vi "MPRL DDA.vi"() -> ()   [LabVIEW 2017]
uses:
  <vilib>/Platform/TimedLoop/XDataNode/timing_clust.ctl
  <vilib>/Platform/TimedLoop/XDataNode/nitl_modes.ctl
  <vilib>/Platform/TimedLoop/XDataNode/wakeup.ctl
  <vilib>/Analysis/Matrix/Datatypes/RealMatrix.ctl
  <vilib>/Analysis/_algsub.llb/Vector Norm Type.ctl
  <vilib>/Analysis/baseanly.llb/A x Vector.vi
  <vilib>/Analysis/baseanly.llb/Real A x B.vi
  <vilib>/Analysis/_algsub.llb/Real Vector Norm.vi
  <vilib>/Analysis/baseanly.llb/Outer Product.vi
  <vilib>/Analysis/baseanly.llb/Real Outer Product.vi
  <vilib>/robotics/Kinematics/Create Lie Group Matrix.vi
  <vilib>/Analysis/7linalg.llb/Create Special Matrix.vi
  <vilib>/Analysis/7linalg.llb/Create Special Real Matrix.vi
  <vilib>/Analysis/Matrix/Numeric/Multiply/Multiply.vi
  <vilib>/Analysis/Matrix/Numeric/Multiply/Multiply - RM,R.vi
  <vilib>/Analysis/Matrix/Numeric/Multiply/Multiply - R,RM.vi
  <vilib>/Analysis/Matrix/Numeric/Add/Add.vi
  <vilib>/Analysis/Matrix/Numeric/Add/Add - RM,RM.vi
  <vilib>/platform/TimedLoop/XDataNode/XDataNode.xnode
  <vilib>/robotics/Kinematics/NI_Kinematics.lvlib
  <vilib>/Analysis/NI_AALBase.lvlib
  <vilib>/Platform/TimedLoop/XDataNode/XDNodeRunTimeDep.lvlib
  <vilib>/Native 3D Graph/xcontrol/3DPC_SurfacePlot.xctl
  <vilib>/Analysis/Matrix/NI_Matrix.lvlib
  <vilib>/Analysis/NI_AALPro.lvlib
  <vilib>/Native 3D Graph/classes/Base Datatype.lvclass
panel:
  out "flag":bool
  out "update":bool
  in  "transition":dbl=10.0
  out "lose":i32
  out "win":i32
  in  "hold":dbl=1.0
  in  "epsilon":dbl=0.1
  out "rpyt":dbl[](array[numeric])=[0.0, -0.7853981633974483, 0.0]
  out "rpyc":dbl[](array[numeric])=[-0.3001584454813599, -0.10145767317616233, -0.18894864398865371]
  out "round":i32=1
  out "chromosome":dbl[](array[numeric])=[0.7617781493855547, 0.4034383827268848, 0.33958668678900183, 0.00421450334971496, 0.9898714458714919, 0.11680136712618072, 0.10145530495952948, 0.8212596957897924, 0.9516478681124503, 0.23533211477594485, 0.6004251129688969, 0.6207875532093379]
  in  "inertia":dbl[](array[numeric])=[0.0, 0.0, 0.0]
  out "torque":dbl[](array[numeric])=[0.0078125, -0.0859375, -0.071441650390625]
  in  "radius":dbl=1.0
  in  "damping":dbl[](array[numeric])=[0.5, 0.5, 0.5]
  in  "theta0":dbl[](array[numeric])=[0.0, 0.0, 0.0] format="%#_15g"
  out "beta2":dbl=0.7460127831658564
  out "v30":dbl[](array[numeric])=[0.5877852522924729, -0.33935797363675174, -0.7344008870614411]
  out "v10":dbl[](array[numeric])=[0.0, 0.6787159472735029, -0.7344008870614411]
  out "v20":dbl[](array[numeric])=[-0.5877852522924731, -0.3393579736367513, -0.7344008870614411]
  out "dt":dbl=0.001
  in  "period":i64=1
  out "v2d":dbl[](array[numeric])=[-0.5634134094645171, -0.44820393165021477, -0.6940306662452641]
  out "v1d":dbl[](array[numeric])=[0.2013119476516629, 0.4244542848654612, -0.882786531270179]
  out "v3d":dbl[](array[numeric])=[0.5852631977932813, -0.6246905878715198, -0.5169416395817887]
  out "thetad":dbl[](array[numeric])=[0.2054876637460845, -0.10844283320485287, 0.2706798683877881] format="%#_15g"
  in  "stop":bool
  out "beta1":dbl=0.9553166181245093
  out "gamma2":dbl=1.2566370614359172
  out "gamma1":dbl=1.5707963267948966
  out "alpha2":dbl=1.5707963267948966
  out "alpha1":dbl=1.5707963267948966
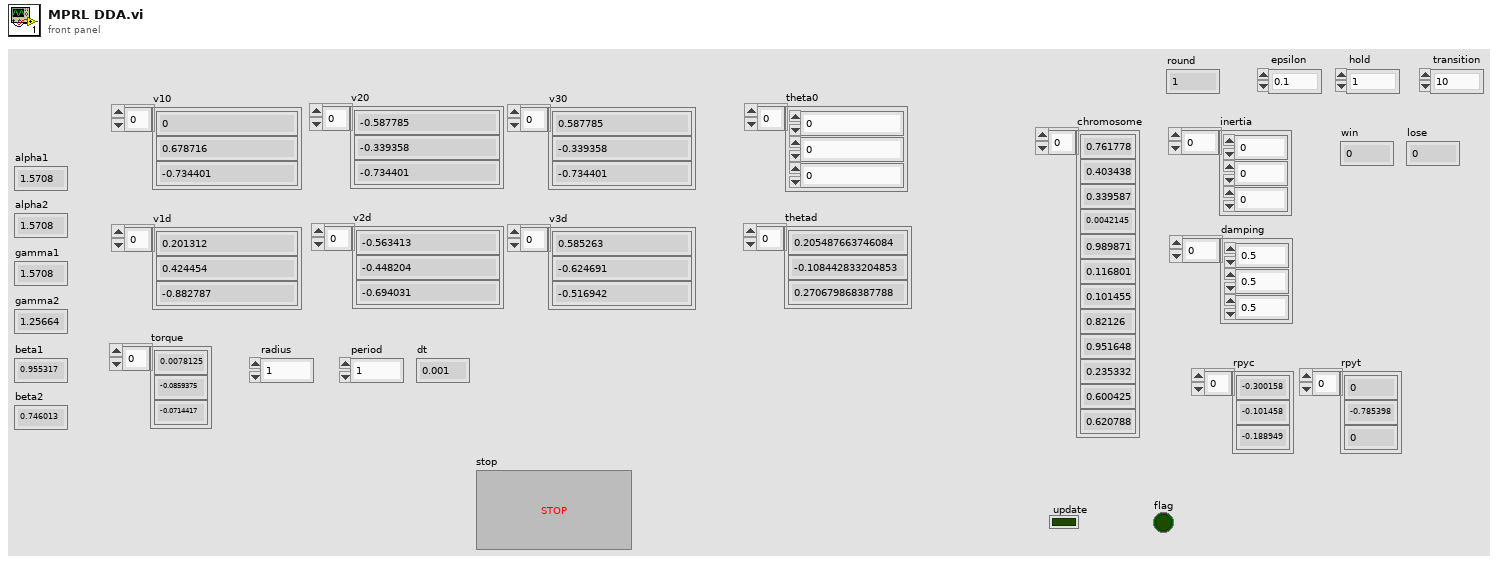
[diagram p1: front panel]
types:
  T1 = typedef "XDNodeRunTimeDep.lvlib/timing_clust.ctl" = cluster{"Expected End [f-1]":u64, "Actual End [f-1]":u64, "Finished Late? [f-1]":bool, "Expected End [i-1]":u64, "Actual End [i-1]":u64, "Finished Late? [i-1]":bool, "Expected Start [i]":u64, "Actual Start [i]":u64, "Expected Start [f]":u64, "Actual Start [f]":u64, "Source Name":string, "Structure Name":string, "Period":i64, "Deadline":i64, "Offset":i64, "Start":i64, "Priority":i32, "Timeout":i32, "Mode":T2, "Wakeup Reason":T3, "Error":errorcluster, "Source Type":string, "Secondary Source Type":string, "Global End Time":u64, "Global Start Time":u64, "Frame Duration":u64, "Iteration Duration":u64, "Assigned CPU":i32, "I/O Scan Engine Mode":u32}
  T2 = typedef "XDNodeRunTimeDep.lvlib/nitl_modes.ctl" = enum32{"No Change", "Process missed periods, maintain original phase", "Discard missed periods, maintain original phase", "Process missed periods, ignore original phase", "Discard missed periods, ignore original phase"}
  T3 = typedef "XDNodeRunTimeDep.lvlib/wakeup.ctl" = enum32{"Normal", "Aborted", "Asynchronous wakeup", "Timing source error", "Timed loop error", "Timeout"}
  T4 = typedef "NI_Matrix.lvlib/RealMatrix.ctl" = dbl[][]
  T5 = typedef "NI_AALPro.lvlib/Vector Norm Type.ctl" = u16
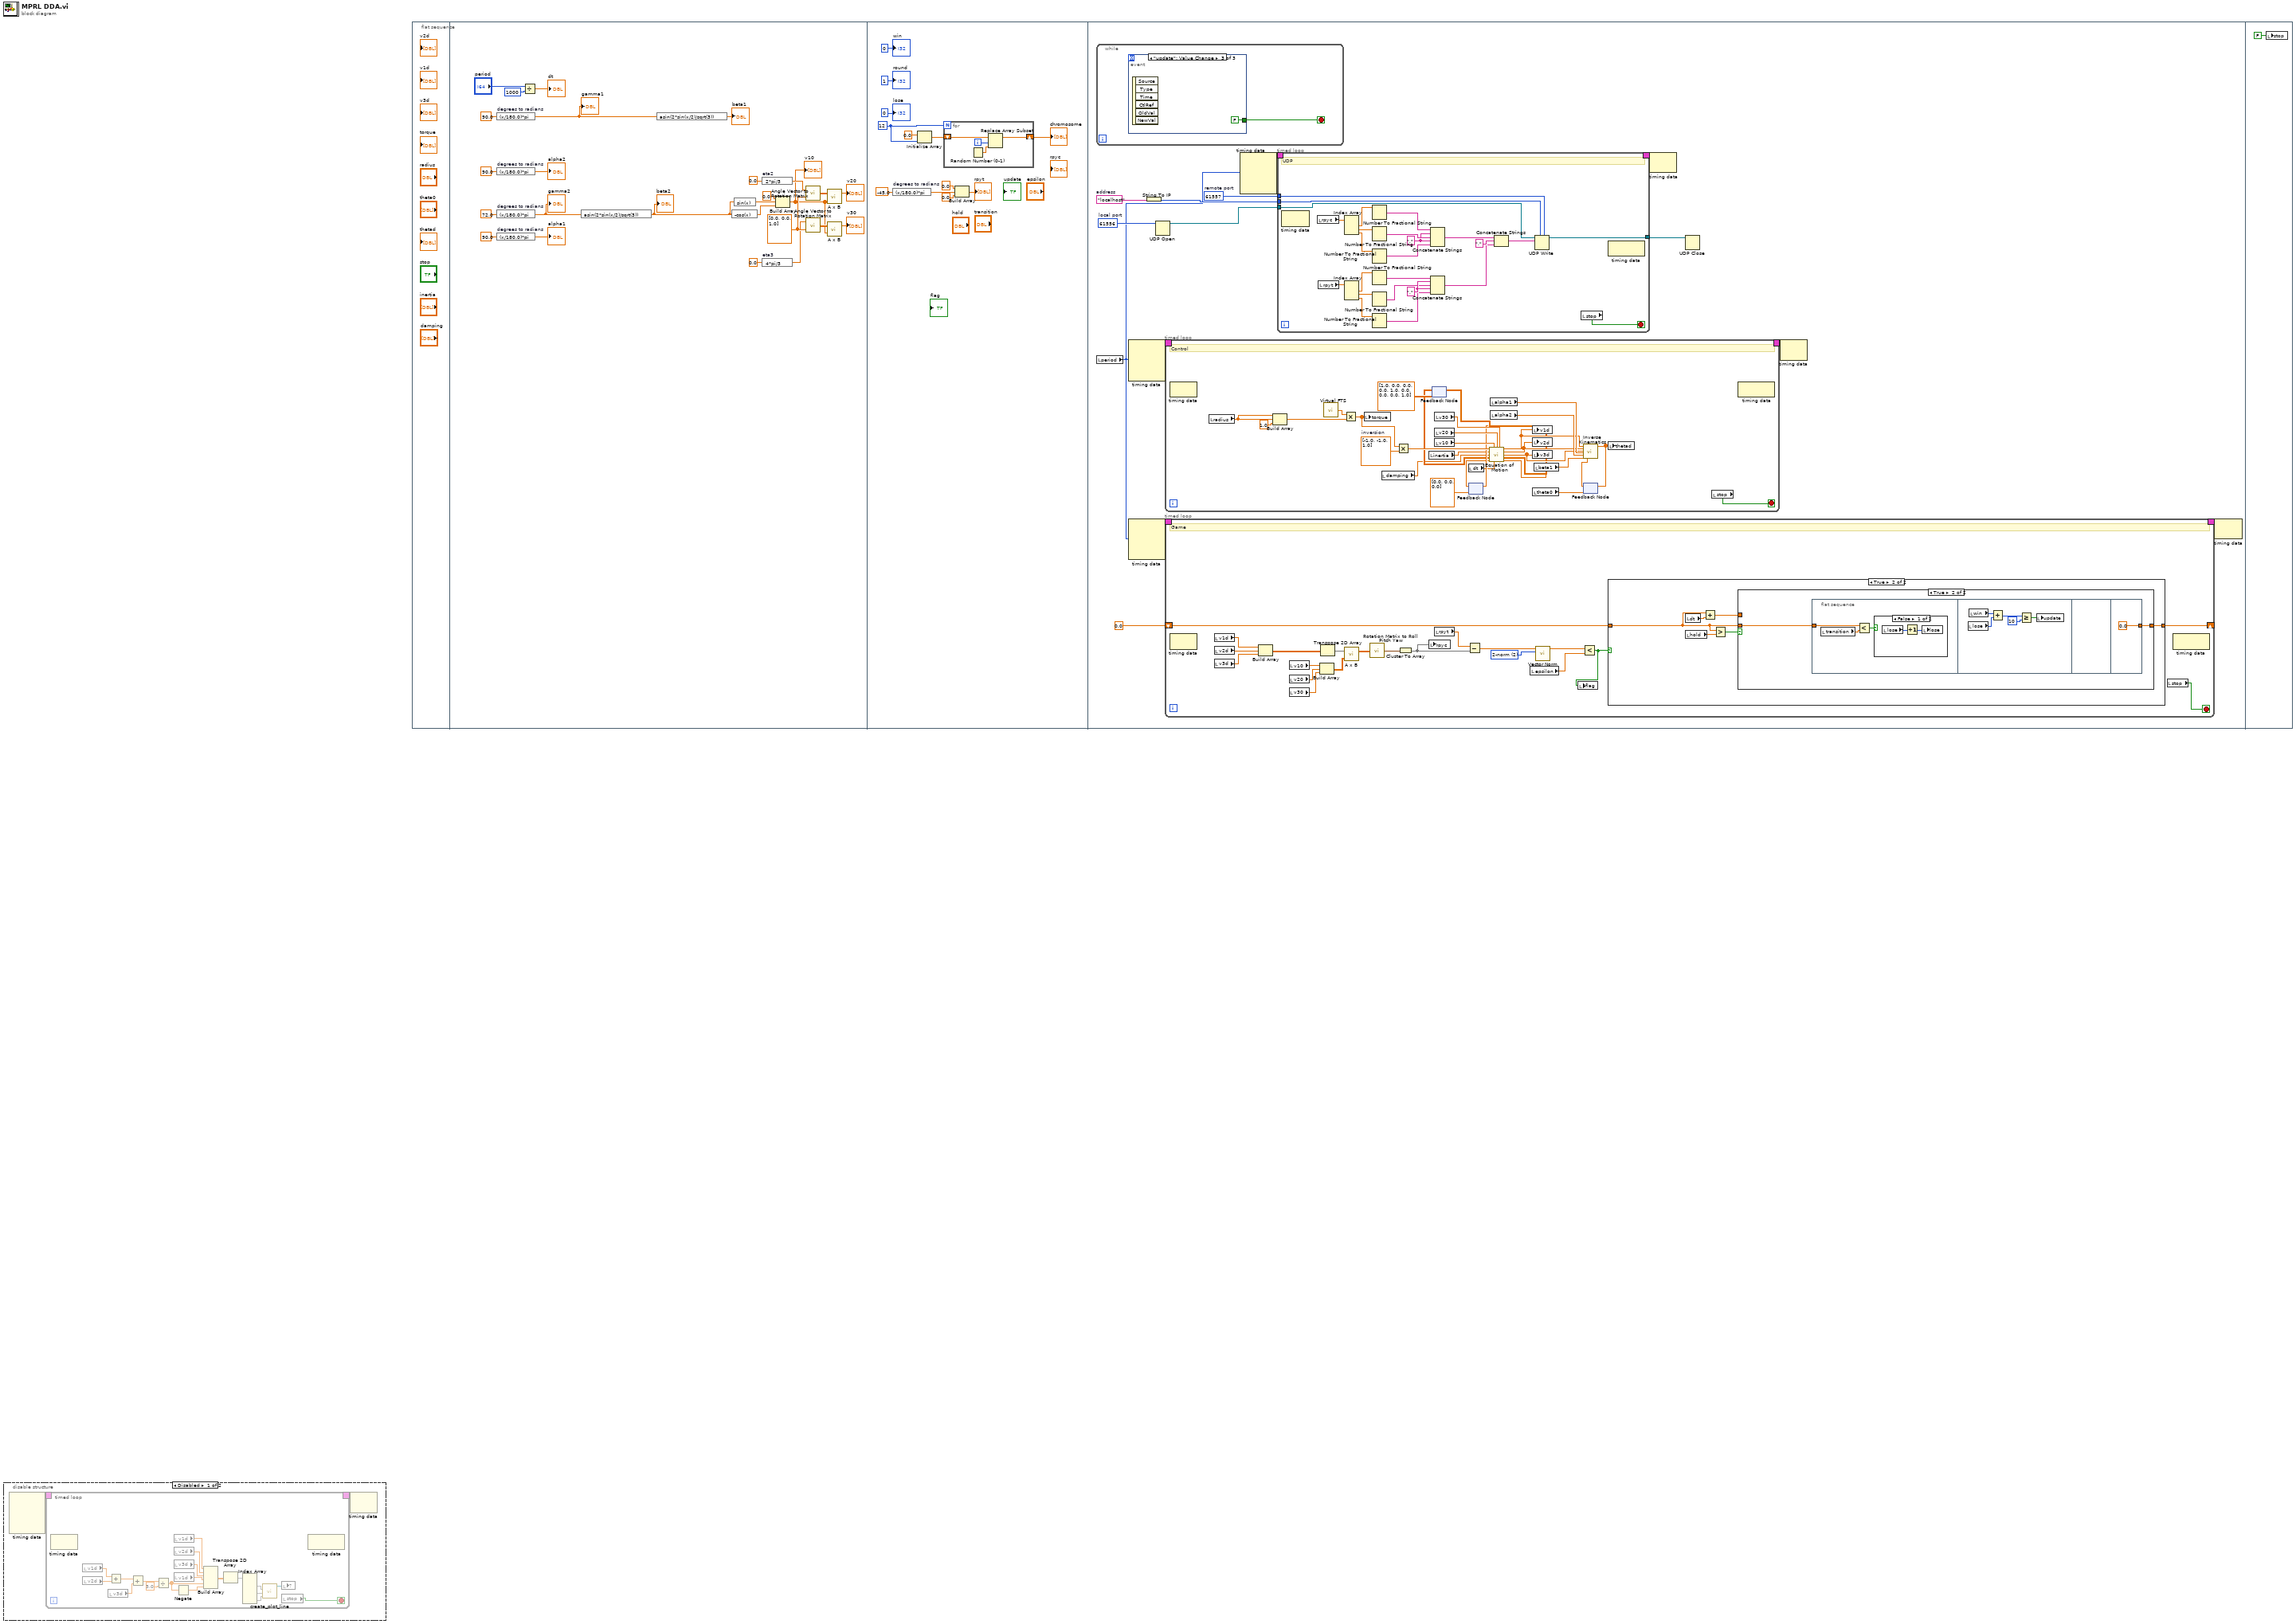
[diagram p0: block diagram]
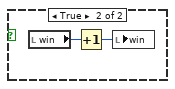
[diagram p5: hidden frame]
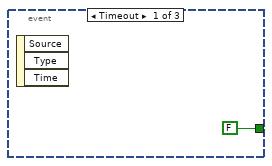
[diagram p6: hidden frame]
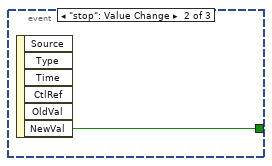
[diagram p7: hidden frame]
diagram:
  n1 = disable-structure shown="Disabled" {
    frame Disabled {
      n2 = node-c288() -> (w2:T1)  [unwired: 4 in]
      n3 = timed-loop {
        timing: w2 -> [_]
        timing-out: [_] -> w1
        stop <- w3 stop-if-true
        n4 = node-c288() -> ()  [unwired: 1 in, 1 out]
        n5 = local read "v1d"() -> (w12:dbl[])
        n6 = local read "v2d"() -> (w11:dbl[])
        n7 = local read "v3d"() -> (w9:dbl[])
        n8 = Add(x=w12, y=w11) -> (x+y=w10:dbl[])
        n9 = Add(x=w10, y=w9) -> (x+y=w8:dbl[])
        n10 = Divide(x=w8, y=3.0) -> (x/y=w6:dbl[])
        n11 = local read "v1d"() -> (w20:dbl[])
        n12 = local read "v2d"() -> (w19:dbl[])
        n13 = local read "v3d"() -> (w18:dbl[])
        n14 = local read "v1d"() -> (w17:dbl[])
        n15 = Negate(x=w6) -> (-x=w5:dbl[])
        n16 = Build Array(w20, w19, w18, w17, w6, w5) -> (w16:dbl[][])
        n17 = Transpose 2D Array(2D array=w16) -> (transposed array=w15:dbl[][])
        n18 = Index Array(array=w15) -> (element #1=w14:dbl[], element #2=w13:dbl[], element #3=w4:dbl[])  [unwired: 6 in]
        n19 = call <vilib>:"create_plot_line.vi"("z vector"=w4, "y vector"=w13, "x vector"=w14) -> ("plots out"=w21:refnum<class "Base Datatype.lvclass">[])  [unwired: 2 in, 6 out]
        n20 = local write item#-1(w21) -> ()
        n21 = local read "stop"() -> (w3:bool)
        n22 = node-c288() -> ()  [unwired: 1 in, 1 out]
      }
      n23 = node-c288(w1) -> ()  [unwired: 1 out]
    }
    frame Enabled {
    }
  }
  n24 = flat-sequence {
    frame #0 {
    }
    frame #1 {
      w48 = dbl[] [0.0, 0.0, 1.0] ("vector")
      # "Kinematics Variables"
      n25 = expression code="(x/180.0)*pi" "degrees to radians"(90.0 ("gamma1")) -> (w32:dbl)
      "gamma1" <- w32
      n26 = expression code="(x/180.0)*pi" "degrees to radians"(90.0 ("alpha2")) -> (→"alpha2":dbl)
      n27 = expression code="(x/180.0)*pi" "degrees to radians"(72.0 ("gamma2")) -> (w30:dbl)
      "gamma2" <- w30
      n28 = expression code="(x/180.0)*pi" "degrees to radians"(90.0 ("alpha1")) -> (→"alpha1":dbl)
      n29 = Divide(x="period", y=i64 1000) -> (x/y=→"dt":dbl)
      n30 = expression code="asin(2*sin(x/2)/sqrt(3))"(w30) -> (w26:dbl)
      "beta2" <- w26
      n31 = expression code="asin(2*sin(x/2)/sqrt(3))"(w32) -> (→"beta1":dbl)
      n32 = expression code="-cos(x)"(w26) -> (w49:dbl)
      n33 = expression code="sin(x)"(w26) -> (w50:dbl)
      n34 = expression code="2*pi/3" "eta2"(0.0) -> (w47:dbl)
      n35 = expression code="4*pi/3" "eta3"(0.0) -> (w46:dbl)
      n36 = Build Array(0.0 ("element"), w50, w49) -> (w41:dbl[])
      "v10" <- w41
      n37 = call <vilib>:"Angle Vector to Rotation Matrix.vi"("vector"=w48, "angle"=w47) -> ("rotation matrix"=w45:T4)
      n38 = call <vilib>:"Angle Vector to Rotation Matrix.vi"("vector"=w48, "angle"=w46) -> ("rotation matrix"=w44:T4)
      n39 = call-poly <vilib>:"A x B.vi"("Vector"=w41, "A"=w45) -> ("A x Vector"=→"v20":dbl[])  [unwired: 1 out]
      n40 = call-poly <vilib>:"A x B.vi"("Vector"=w41, "A"=w44) -> ("A x Vector"=→"v30":dbl[])  [unwired: 1 out]
    }
    frame #2 {
      w61 = 12
      n41 = expression code="(x/180.0)*pi" "degrees to radians"(-45.0 ("alpha1")) -> (w57:dbl)
      n42 = Initialize Array(0.0 ("element"), w61) -> (w63:dbl[])
      n43 = for {
        N: w61 -> [_]
        shift-right: [w64] -> w60
        shift-left: w63 -> [w67]
        i -> [w66]
        n44 = Random Number (0-1)() -> (number: 0 to 1=w65:dbl)
        n45 = Replace Array Subset(array=w67, new element=w65, index=w66) -> (w64:dbl[])
      }
      "chromosome" <- w60
      n46 = Build Array(0.0 ("element"), w57, 0.0 ("element")) -> (→"rpyt":dbl[])
      "round" <- 1
      "win" <- 0 ("win")
      "lose" <- 0 ("lose")
    }
    frame #3 {
      w72 = "localhost"  # address
      w74 = u16 61557  # remote port
      w77 = u16 61556  # local port
      # "FK/IK"
      n47 = while {
        stop <- w132 stop-if-true
        n48 = event shown="[2] \"update\": Value Change" {
          selector: _ -> [_ _ _]
          dyn-events: _ -> [_ _ _]
          timeout: _ -> [_ _ _]
          tunnel: [FALSE ("NewVal") w134 FALSE ("NewVal")] -> w132
          event Timeout {
            n49 = event-data() -> ()  [unwired: 1 in, 3 out]
          }
          event "stop": Value Change {
            n50 = event-data() -> ("NewVal"=w134:bool)  [unwired: 1 in, 5 out]
          }
          event "update": Value Change {
            n51 = event-data() -> ()  [unwired: 1 in, 6 out]
          }
        }
      }
      n52 = local read "period"() -> (w68:i64)
      n53 = node-c288(w68) -> (w81:T1)  [unwired: 3 in]
      n54 = node-c288(w68) -> (w71:T1)  [unwired: 3 in]
      n55 = String To IP(1:w72) -> (0:w73:u32)
      n56 = UDP Open(11:w77) -> (port=w76:refnum<k16>)  [unwired: 4 in, 2 out]
      n57 = timed-loop "Timed Loop" {
        timing: w81 -> [_]
        timing-out: [_] -> w80
        stop <- w195 stop-if-true
        w179 = dbl[] [-1.0, -1.0, 1.0]  # inversion
        # "Control"
        n58 = node-c288() -> ()  [unwired: 1 in, 1 out]
        n59 = local read "radius"() -> (w176:dbl)
        n60 = Build Array(w176, w176, 1.0 ("element")) -> (w173:dbl[])
        n61 = call "Virtual FTS.vi"() -> ("value"=w174:dbl[])
        n62 = Multiply(x=w174, y=w173) -> (x*y=w172:dbl[])
        n63 = local write "torque"(w172) -> ()
        n64 = local read "damping"() -> (w167:dbl[])
        n65 = Multiply(x=w172, y=w179) -> (x*y=w180:dbl[])
        n66 = local read "inertia"() -> (w168:dbl[])
        n67 = feedback #1(T4 [[1.0, 0.0, 0.0], [0.0, 1.0, 0.0], [0.0, 0.0, 1.0]] ("R'")) -> (w169:T4)
        n68 = local read "v30"() -> (w181:dbl[])
        n69 = local read "v20"() -> (w182:dbl[])
        n70 = local read "v10"() -> (w183:dbl[])
        n71 = local read "dt"() -> (w171:dbl)
        n72 = feedback #2(dbl[] [0.0, 0.0, 0.0] ("flow'")) -> (w170:dbl[])
        n73 = call "Equation of Motion.vi"("torque"=w180, "v10"=w183, "v20"=w182, "v30"=w181, "inertia"=w168, "damping"=w167, "R"=w169, "omega"=w170, "dt"=w171) -> ("v1d"=w188:dbl[], "v2d"=w187:dbl[], "v3d"=w186:dbl[], "R'"=w185:T4, "omega'"=w178:dbl[])  [unwired: 2 in]
        n74 = feedback-in #1(w185) -> ()
        n75 = feedback-in #2(w178) -> ()
        n76 = local read "alpha1"() -> (w190:dbl)
        n77 = local read "alpha2"() -> (w191:dbl)
        n78 = local write "v1d"(w188) -> ()
        n79 = local write "v2d"(w187) -> ()
        n80 = local write "v3d"(w186) -> ()
        n81 = local read "theta0"() -> (w193:dbl[])
        n82 = local read "beta1"() -> (w192:dbl)
        n83 = feedback #3(w193) -> (w194:dbl[])
        n84 = call "Inverse Kinematics.vi"("v1"=w188, "v2"=w187, "v3"=w186, "alpha1"=w190, "alpha2"=w191, "beta1"=w192, "theta"=w194) -> ("theta'"=w189:dbl[])  [unwired: 12 in]
        n85 = feedback-in #3(w189) -> ()
        n86 = local write "thetad"(w189) -> ()
        n87 = local read "stop"() -> (w195:bool)
        n88 = node-c288() -> ()  [unwired: 1 in, 1 out]
      }
      n89 = timed-loop "Timed Loop" {
        timing: w71 -> [_]
        timing-out: [_] -> w70
        shift-right: [w97] -> _
        shift-left: 0.0 -> [w96]
        stop <- w82 stop-if-true
        w99 = T5 2 items=["1-norm"=1, "2-norm"=2, "Inf-norm"=3, "-Inf-norm"=4, "User Defined"=5] ("norm type")
        # "Game"
        n90 = node-c288() -> ()  [unwired: 1 in, 1 out]
        n91 = local read "v1d"() -> (w85:dbl[])
        n92 = local read "v2d"() -> (w86:dbl[])
        n93 = local read "v3d"() -> (w87:dbl[])
        n94 = Build Array(w85, w86, w87) -> (w91:dbl[][])
        n95 = local read "v10"() -> (w90:dbl[])
        n96 = local read "v20"() -> (w89:dbl[])
        n97 = local read "v30"() -> (w88:dbl[])
        n98 = Build Array(w90, w89, w88) -> (w93:dbl[][])
        n99 = Transpose 2D Array(2D array=w91) -> (transposed array=w92:dbl[][])
        n100 = call-poly <vilib>:"A x B.vi"("B"=w93, "A"=w92) -> ("A x B"=w94:T4)  [unwired: 1 out]
        n101 = call <vilib>:"Rotation Matrix to Roll Pitch Yaw.vi"("rotation matrix"=w94) -> ("angles"=w95:cluster{"roll":dbl, "pitch":dbl, "yaw":dbl})
        n102 = Cluster To Array(cluster=w95) -> (array=w84:dbl[])
        n103 = local write "rpyc"(w84) -> ()
        n104 = local read "rpyt"() -> (w102:dbl[])
        n105 = Subtract(x=w102, y=w84) -> (x-y=w98:dbl[])
        n106 = local read "epsilon"() -> (w101:dbl)
        n107 = call-poly <vilib>:"Vector Norm.vi"("norm type"=w99, "Input Vector"=w98) -> ("norm"=w100:dbl)  [unwired: 8 in, 1 out]
        n108 = Less?(x=w100, y=w101) -> (x < y?=w83:bool)
        n109 = local write "flag"(w83) -> ()
        n110 = case shown="True" w83 {
          tunnel: w96 -> [w103 w106]
          tunnel: [w103 w104] -> w97
          frame False {
          }
          frame True {
            n111 = local read "dt"() -> (w109:dbl)
            n112 = local read "hold"() -> (w108:dbl)
            n113 = Add(x=w106, y=w109) -> (x+y=w105:dbl)
            n114 = Greater?(x=w106, y=w108) -> (0:w107:bool)
            n115 = case shown="True" w107 {
              tunnel: w106 -> [_ w112]
              tunnel: w105 -> [w110 _]
              tunnel: [w110 w111] -> w104
              frame False {
              }
              frame True {
                n116 = flat-sequence {
                  tunnel: w112 -> [w113]
                  tunnel: [0.0] -> w111
                  frame #0 {
                    n117 = local read "transition"() -> (w115:dbl)
                    n118 = Less?(x=w113, y=w115) -> (x < y?=w114:bool)
                    n119 = case shown="False" w114 {
                      frame False {
                        n120 = local read "lose"() -> (w117:i32)
                        n121 = Increment(x=w117) -> (x+1=w116:i32)
                        n122 = local write "lose"(w116) -> ()
                      }
                      frame True {
                        n123 = local read "win"() -> (w119:i32)
                        n124 = Increment(x=w119) -> (x+1=w118:i32)
                        n125 = local write "win"(w118) -> ()
                      }
                    }
                  }
                  frame #1 {
                    n126 = local read "lose"() -> (w123:i32)
                    n127 = local read "win"() -> (w124:i32)
                    n128 = Add(x=w124, y=w123) -> (x+y=w122:i32)
                    n129 = Greater Or Equal?(x=w122, y=10) -> (x >= y?=w120:bool)
                    n130 = local write "update"(w120) -> ()
                  }
                  frame #2 {
                  }
                  frame #3 {
                  }
                }
              }
            }
          }
        }
        n131 = local read "stop"() -> (w82:bool)
        n132 = node-c288() -> ()  [unwired: 1 in, 1 out]
      }
      n133 = node-c288(w68) -> (w79:T1)  [unwired: 3 in]
      n134 = timed-loop "Timed Loop" {
        timing: w79 -> [_]
        timing-out: [_] -> w78
        tunnel: w76 -> [w160]
        tunnel: [w159] -> w75
        tunnel: w74 -> [w151]
        tunnel: w73 -> [w150]
        stop <- w138 stop-if-true
        w149 = "," ("string")
        w152 = "," ("string")
        # "UDP"
        n135 = node-c288() -> ()  [unwired: 1 in, 1 out]
        n136 = local read "rpyc"() -> (w136:dbl[])
        n137 = local read "rpyt"() -> (w137:dbl[])
        n138 = Index Array(array=w136) -> (element #1=w158:dbl, element #2=w157:dbl, element #3=w156:dbl)  [unwired: 3 in]
        n139 = Index Array(array=w137) -> (element #1=w145:dbl, element #2=w144:dbl, element #3=w143:dbl)  [unwired: 3 in]
        n140 = Number To Fractional String(number=w158) -> (F-format string=w155:string)  [unwired: 3 in]
        n141 = Number To Fractional String(number=w157) -> (F-format string=w154:string)  [unwired: 3 in]
        n142 = Number To Fractional String(number=w156) -> (F-format string=w153:string)  [unwired: 3 in]
        n143 = Number To Fractional String(number=w145) -> (F-format string=w146:string)  [unwired: 3 in]
        n144 = Number To Fractional String(number=w144) -> (F-format string=w147:string)  [unwired: 3 in]
        n145 = Number To Fractional String(number=w143) -> (F-format string=w148:string)  [unwired: 3 in]
        n146 = Concatenate Strings(w155, w152, w154, w152, w153) -> (w141:string)
        n147 = Concatenate Strings(w146, w149, w147, w149, w148) -> (w140:string)
        n148 = Concatenate Strings(w141, "," ("string"), w140) -> (w139:string)
        n149 = UDP Write(address=w150, port or service name=w151, connection ID=w160, data in=w139) -> (3:w159:refnum<k16>)  [unwired: 2 in, 1 out]
        n150 = local read "stop"() -> (w138:bool)
        n151 = node-c288() -> ()  [unwired: 1 in, 1 out]
      }
      n152 = node-c288(w78) -> ()  [unwired: 1 out]
      n153 = UDP Close(connection ID=w75) -> ()  [unwired: 1 in, 2 out]
      n154 = node-c288(w80) -> ()  [unwired: 1 out]
      n155 = node-c288(w70) -> ()  [unwired: 1 out]
    }
    frame #4 {
      n156 = local write "stop"(FALSE ("stop")) -> ()
    }
  }
